vi "Feature_Names.vi"(8 "error in (no error)":errorcluster caption="entrée d'erreur (pas d'erreur)", 11 "Load_Wine en entrée":refnum<class "Load_Wine.lvclass">) -> (0 "error out":errorcluster caption="sortie d'erreur", 3 "Load_Wine en sortie":refnum<class "Load_Wine.lvclass">)   [LabVIEW 2020, in "Load_Wine.lvclass"]
uses:
  Load_Wine.lvclass
  Load_Wine.lvclass/Load_Wine.ctl
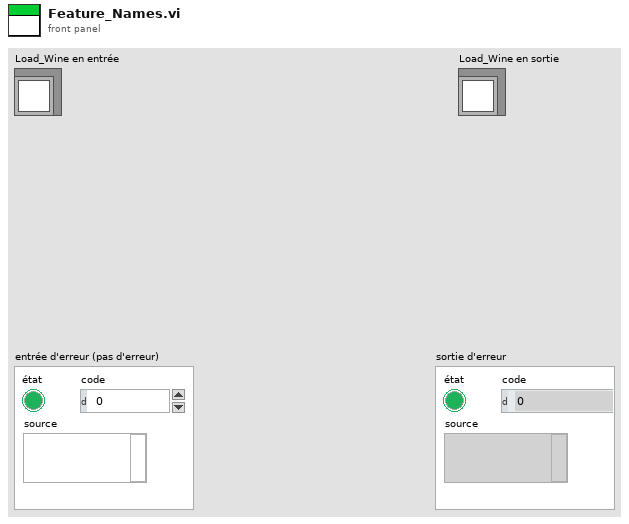
[diagram p1: front panel]
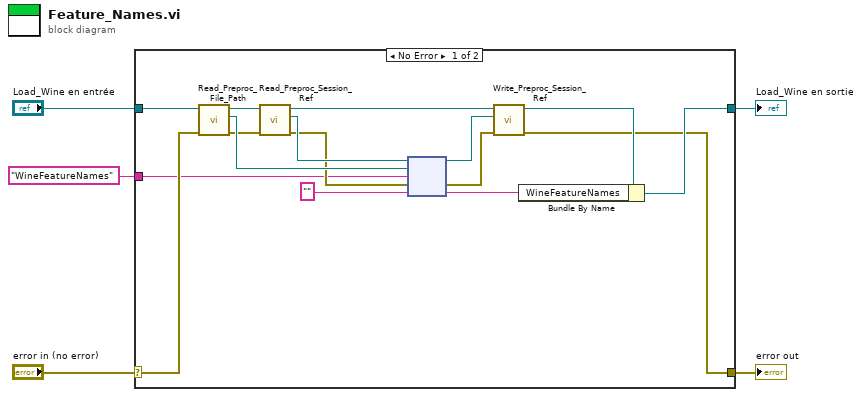
[diagram p0: block diagram]
diagram:
  n1 = case shown="No Error" "error in (no error)" {
    selector: "error in (no error)" -> [w7 w23]
    tunnel: [w8 w23] -> w4
    tunnel: [w9 w22] -> w2
    tunnel: "Load_Wine en entrée" -> [w10 w22]
    tunnel: "WineFeatureNames" -> [w6 _]
    frame No Error {
      n2 = call-dynamic "Read_Preproc_File_Path.vi"("error in (no error)"=w7, "Python in"=w10) -> ("error out"=w16:errorcluster, "File_Path"=w19:path, "Python out"=w21:refnum<class "Load_Wine.lvclass">)  [unwired: 7 in]
      n3 = call-dynamic "Read_Preproc_Session_Ref.vi"("error in (no error)"=w16, "Python in"=w21) -> ("error out"=w17:errorcluster, "Session_ref"=w18:refnum<k35>, "Python out"=w20:refnum<class "Load_Wine.lvclass">)  [unwired: 7 in]
      n4 = node(w18, w19, w6, w17, "") -> (w13:refnum<k35>, w15:errorcluster, w12:string)  [unwired: 2 out]
      n5 = call-dynamic "Write_Preproc_Session_Ref.vi"("error in (no error)"=w15, "Session_ref"=w13, "Python in"=w20) -> ("error out"=w8:errorcluster, "Python out"=w11:refnum<class "Load_Wine.lvclass">)  [unwired: 7 in]
      n6 = Bundle By Name(cluster=w11, "WineFeatureNames"=w12) -> (w9:refnum<class "Load_Wine.lvclass">)
    }
    frame Error {
    }
  }
  "error out" <- w4
  "Load_Wine en sortie" <- w2
